vi "GenBinArrays_FASTSCAN.vi"(4 "Pixels Per Line":dbl=1024.0, 5 "FPGA Acquisition Clock Rate (MHz)":dbl=200.0, 6 "Collection Percent (%)":dbl=64.0, 7 "Scan Rate (kHz)":dbl=16.0) -> (0 "Reported Parameters":T1, 1 "Normalization Array":sgl[](array[numeric]), 2 "Pre Binned Counts (x100)":u32[](array[numeric]), 3 "FPGA Bin Edges":bool[](array[boolean]))   [LabVIEW 2014]
panel:
  out "Average Pixel Dwell Time":dbl
  out "FPGA Sampling Period (ns)":dbl
  out "Counting Period Edges (ns)":dbl[](array[numeric]) format="%#_10g"
  out "Normalized Scan Start Position":dbl
  out "Normalized Scan End Position":dbl
  out "Stop Time (us)":dbl
  out "Start Time (us)":dbl
  out "Samples Per Counting Period":i32
  out "Counting Period (us)":dbl
  # "Note that at transition points the fractional photons have been combined for data packing."
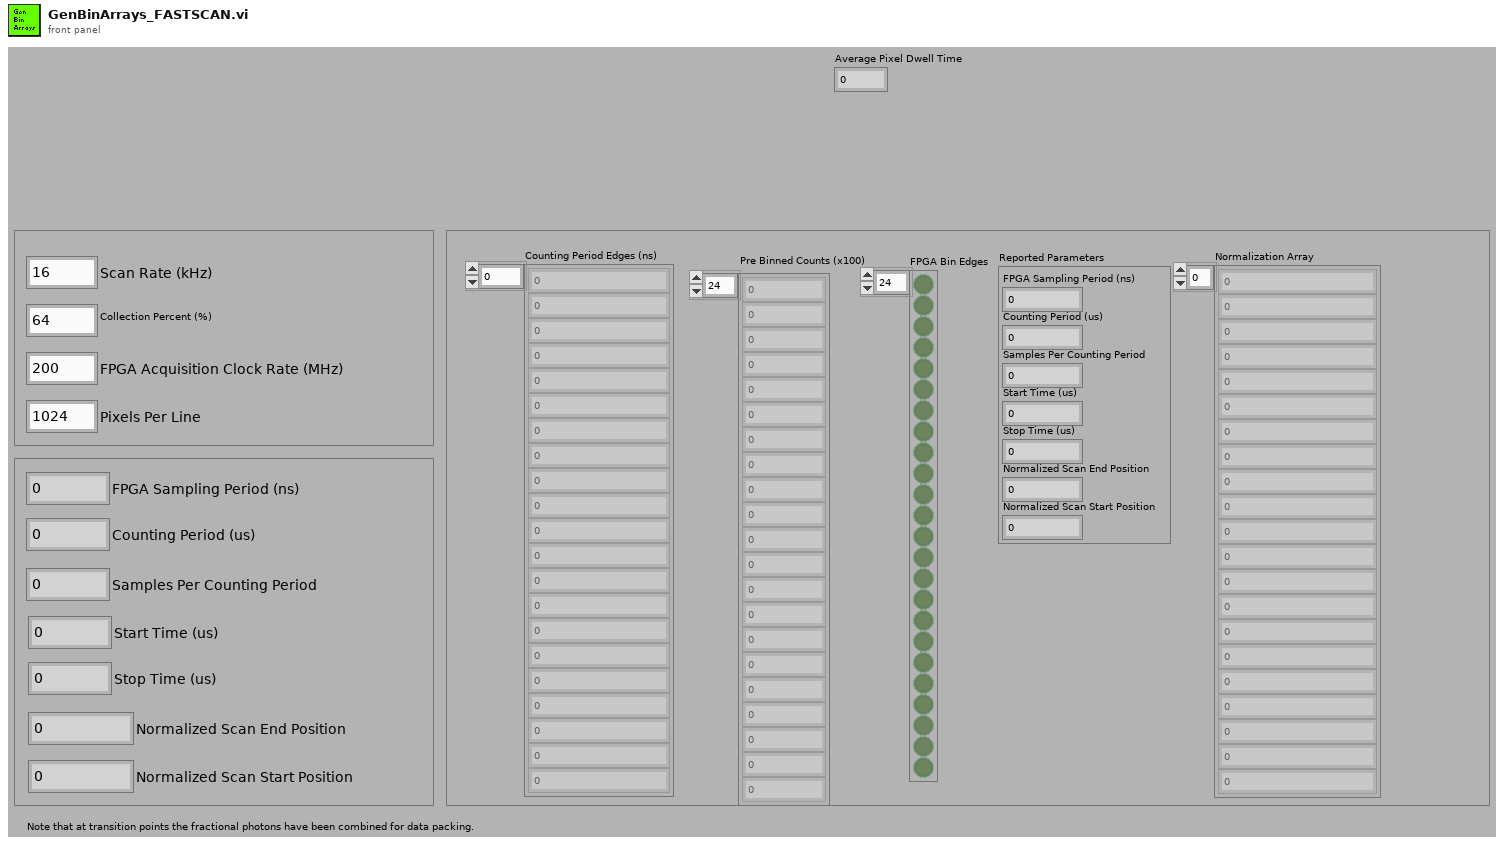
[diagram p1: front panel]
types:
  T1 = cluster{"FPGA Sampling Period (ns)":dbl, "Counting Period (us)":dbl, "Samples Per Counting Period":i32, "Start Time (us)":dbl, "Stop Time (us)":dbl, "Normalized Scan End Position":dbl, "Normalized Scan Start Position":dbl}
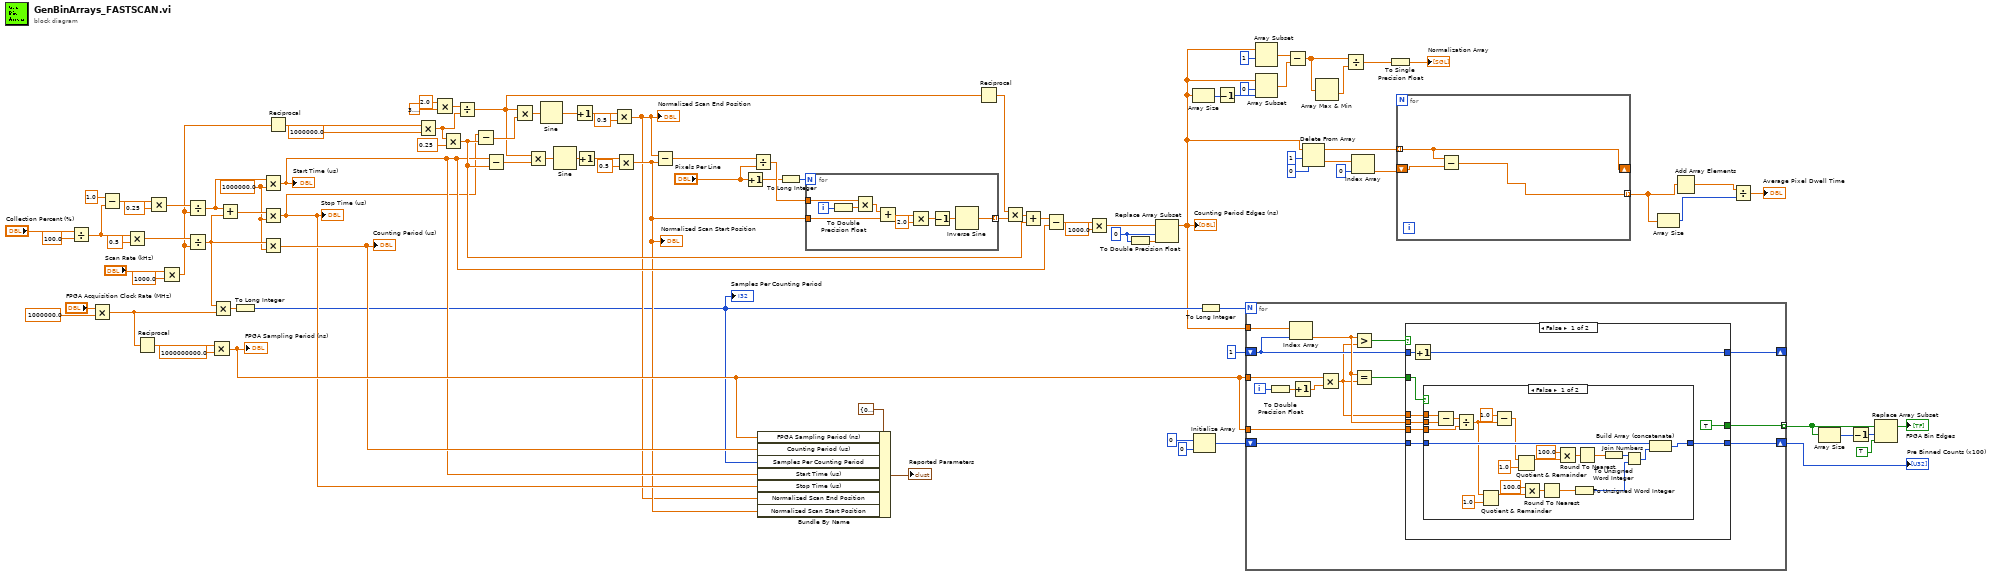
[diagram p0: block diagram]
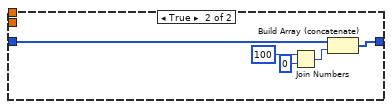
[diagram p2: hidden frame]
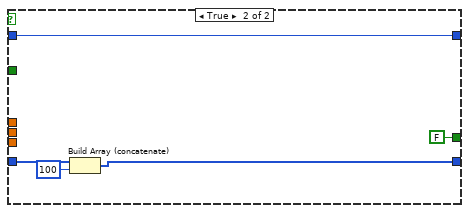
[diagram p3: hidden frame]
diagram:
  w48 = 0 ("index")
  w81 = 1000000.0 ("y")
  n1 = Divide(x="Collection Percent (%)", y=100.0) -> (x/y=w90:dbl)
  n2 = Multiply(x="FPGA Acquisition Clock Rate (MHz)", y=1000000.0) -> (x*y=w47:dbl)
  n3 = Subtract(x=1.0, y=w90) -> (x-y=w89:dbl)
  n4 = Multiply(x=w90, y=0.5) -> (x*y=w92:dbl)
  n5 = Reciprocal(x=w47) -> (1/x=w46:dbl)
  n6 = Multiply(x=w89, y=0.25) -> (x*y=w87:dbl)
  n7 = Multiply(x="Scan Rate (kHz)", y=1000.0) -> (x*y=w62:dbl)
  n8 = Divide(x=w87, y=w62) -> (x/y=w71:dbl)
  n9 = Divide(x=w92, y=w62) -> (x/y=w83:dbl)
  n10 = Multiply(x=w46, y=1000000000.0) -> (x*y=w33:dbl)
  "FPGA Sampling Period (ns)" <- w33
  n11 = Multiply(x=w83, y=w47) -> (x*y=w31:dbl)
  n12 = Add(x=w71, y=w83) -> (x+y=w82:dbl)
  n13 = To Long Integer(number=w31) -> (32bit integer=w26:i32)
  "Samples Per Counting Period" <- w26
  n14 = Multiply(x=w71, y=w81) -> (x*y=w30:dbl)
  "Start Time (us)" <- w30
  n15 = Multiply(x=w82, y=w81) -> (x*y=w29:dbl)
  "Stop Time (us)" <- w29
  n16 = Multiply(x=w83, y=w81) -> (x*y=w32:dbl)
  "Counting Period (us)" <- w32
  n17 = Reciprocal(x=w62) -> (1/x=w69:dbl)
  n18 = Multiply(x=w69, y=1000000.0) -> (x*y=w68:dbl)
  n19 = Multiply(x=2.0 ("y"), y=3.141592653589793) -> (x*y=w77:dbl)
  n20 = Multiply(x=w68, y=0.25) -> (x*y=w54:dbl)
  n21 = Divide(x=w77, y=w68) -> (x/y=w58:dbl)
  n22 = Subtract(x=w29, y=w54) -> (x-y=w76:dbl)
  n23 = Subtract(x=w30, y=w54) -> (x-y=w63:dbl)
  n24 = Multiply(x=w58, y=w76) -> (x*y=w75:dbl)
  n25 = Multiply(x=w58, y=w63) -> (x*y=w64:dbl)
  n26 = Sine(x=w75) -> (sin(x)=w74:dbl)
  n27 = Sine(x=w64) -> (sin(x)=w65:dbl)
  n28 = Increment(x=w74) -> (x+1=w73:dbl)
  n29 = Increment(x=w65) -> (x+1=w66:dbl)
  n30 = Multiply(x=w73, y=0.5) -> (x*y=w27:dbl)
  "Normalized Scan End Position" <- w27
  n31 = Multiply(x=w66, y=0.5) -> (x*y=w28:dbl)
  "Normalized Scan Start Position" <- w28
  n32 = Subtract(x=w27, y=w28) -> (x-y=w61:dbl)
  n33 = Increment(x="Pixels Per Line") -> (x+1=w35:dbl)
  n34 = Divide(x=w61, y="Pixels Per Line") -> (x/y=w60:dbl)
  n35 = Bundle By Name(cluster=T1 {"FPGA Sampling Period (ns)"=0.0, "Counting Period (us)"=0.0, "Samples Per Counting Period"=0, "Start Time (us)"=0.0, "Stop Time (us)"=0.0, "Normalized Scan End Position"=0.0, "Normalized Scan Start Position"=0.0}, "FPGA Sampling Period (ns)"=w33, "Counting Period (us)"=w32, "Samples Per Counting Period"=w26, "Start Time (us)"=w30, "Stop Time (us)"=w29, "Normalized Scan End Position"=w27, "Normalized Scan Start Position"=w28) -> (→"Reported Parameters":T1)
  n36 = To Long Integer(number=w35) -> (32bit integer=w59:i32)
  n37 = for {
    N: w59 -> [_]
    tunnel: w28 -> [w106]
    tunnel: w60 -> [w105]
    tunnel: [w98] -> w57 mode=indexing
    i -> [w104]
    n38 = To Double Precision Float(number=w104) -> (double precision float=w103:dbl)
    n39 = Multiply(x=w105, y=w103) -> (x*y=w102:dbl)
    n40 = Add(x=w102, y=w106) -> (x+y=w97:dbl)
    n41 = Multiply(x=w97, y=2.0) -> (x*y=w100:dbl)
    n42 = Decrement(x=w100) -> (x-1=w99:dbl)
    n43 = Inverse Sine(1:w99) -> (0:w98:dbl)
  }
  n44 = Reciprocal(x=w58) -> (1/x=w56:dbl)
  n45 = Multiply(x=w56, y=w57) -> (x*y=w55:dbl[])
  n46 = Add(x=w55, y=w54) -> (x+y=w53:dbl[])
  n47 = Subtract(x=w53, y=w30) -> (x-y=w52:dbl[])
  n48 = Multiply(x=w52, y=1000.0) -> (x*y=w50:dbl[])
  n49 = To Double Precision Float(number=w48) -> (double precision float=w49:dbl)
  n50 = Replace Array Subset(array=w50, new element=w49, index=w48) -> (w11:dbl[])
  "Counting Period Edges (ns)" <- w11
  n51 = Array Size(array=w11) -> (size(s)=w24:i32)
  n52 = Initialize Array(u32 0 ("element"), 0 ("dimension size")) -> (w41:u32[])
  n53 = To Long Integer(number=w26) -> (32bit integer=w25:i32)
  n54 = Decrement(x=w24) -> (x-1=w22:i32)
  n55 = for {
    N: w25 -> [_]
    tunnel: w33 -> [w118]
    tunnel: w11 -> [w121]
    shift-right: [w109] -> _
    shift-left: 1 ("index") -> [w110]
    shift-right: [w114] -> w13
    shift-left: w41 -> [w115]
    tunnel: w33 -> [w112]
    tunnel: [w108] -> w37 mode=indexing
    i -> [w119]
    n56 = To Double Precision Float(number=w119) -> (double precision float=w120:dbl)
    n57 = Index Array(array=w121, index=w110) -> (element=w113:dbl)
    n58 = Increment(x=w120) -> (x+1=w117:dbl)
    n59 = Multiply(x=w118, y=w117) -> (x*y=w107:dbl)
    n60 = Greater?(x=w113, y=w107) -> (0:w116:bool)
    n61 = Equal?(x=w113, y=w107) -> (x = y?=w111:bool)
    n62 = case shown="False" w116 {
      tunnel: w115 -> [w127 w162]
      tunnel: [w126 w160] -> w114
      tunnel: [TRUE FALSE] -> w108
      tunnel: w107 -> [w130 _]
      tunnel: w113 -> [w129 _]
      tunnel: w112 -> [w128 _]
      tunnel: w111 -> [w122 _]
      tunnel: w110 -> [w124 w158]
      tunnel: [w123 w158] -> w109
      frame False {
        n63 = Increment(x=w124) -> (x+1=w123:i32)
        n64 = case shown="False" w122 {
          tunnel: w130 -> [w151 _]
          tunnel: w129 -> [w150 _]
          tunnel: w128 -> [w149 _]
          tunnel: w127 -> [w147 w157]
          tunnel: [w146 w156] -> w126
          frame False {
            n65 = Subtract(x=w151, y=w150) -> (x-y=w152:dbl)
            n66 = Divide(x=w152, y=w149) -> (x/y=w141:dbl)
            n67 = Quotient & Remainder(x=w141, y=1.0) -> (x-y*floor(x/y)=w143:dbl)  [unwired: 1 out]
            n68 = Subtract(x=1.0, y=w141) -> (x-y=w134:dbl)
            n69 = Quotient & Remainder(x=w134, y=1.0) -> (x-y*floor(x/y)=w137:dbl)  [unwired: 1 out]
            n70 = Multiply(x=100.0, y=w143) -> (x*y=w145:dbl)
            n71 = Round To Nearest(number=w145) -> (nearest integer value=w140:dbl)
            n72 = Multiply(x=100.0, y=w137) -> (x*y=w135:dbl)
            n73 = To Unsigned Word Integer(number=w140) -> (unsigned 16bit integer=w132:u16)
            n74 = Round To Nearest(number=w135) -> (nearest integer value=w139:dbl)
            n75 = To Unsigned Word Integer(number=w139) -> (unsigned 16bit integer=w133:u16)
            n76 = Join Numbers(hi=w133, lo=w132) -> ((hi.lo)=w131:u32)
            n77 = Build Array (concatenate)(w147, w131) -> (w146:u32[])
          }
          frame True {
            n78 = Join Numbers(hi=u16 100, lo=u16 0) -> ((hi.lo)=w153:u32)
            n79 = Build Array (concatenate)(w157, w153) -> (w156:u32[])
          }
        }
      }
      frame True {
        n80 = Build Array (concatenate)(w162, u32 100) -> (w160:u32[])
      }
    }
  }
  "Pre Binned Counts (x100)" <- w13
  n81 = Array Subset(array=w11, index=1) -> (w20:dbl[])  [unwired: 1 in]
  n82 = Array Subset(array=w11, index=0, length=w22) -> (w19:dbl[])
  n83 = Subtract(x=w20, y=w19) -> (x-y=w18:dbl[])
  n84 = Delete From Array(array=w11, length=1, index=0) -> (deleted portion=w8:dbl[], array with subset deleted=w6:dbl[])
  n85 = Array Max & Min(array=w18) -> (min value=w17:dbl)  [unwired: 3 out]
  n86 = Divide(x=w18, y=w17) -> (x/y=w16:dbl[])
  n87 = Index Array(array=w8, index=0) -> (element=w5:dbl)
  n88 = To Single Precision Float(number=w16) -> (single precision float=→"Normalization Array":sgl[])
  n89 = for {
    tunnel: w6 -> [w165] mode=indexing
    shift-right: [w165] -> _
    shift-left: w5 -> [w164]
    tunnel: [w163] -> w4 mode=indexing
    n90 = Subtract(x=w165, y=w164) -> (x-y=w163:dbl)
  }
  n91 = Array Size(array=w4) -> (size(s)=w2:i32)
  n92 = Add Array Elements(numeric array=w4) -> (sum=w3:dbl)
  n93 = Divide(x=w3, y=w2) -> (x/y=→"Average Pixel Dwell Time":dbl)
  n94 = Array Size(array=w37) -> (size(s)=w40:i32)
  n95 = Decrement(x=w40) -> (x-1=w39:i32)
  n96 = Replace Array Subset(array=w37, new element=TRUE, index=w39) -> (→"FPGA Bin Edges":bool[])
